vi "Event Receive.vi"(11 "jettl Event Actor in":refnum<class "jettl Event Actor.lvclass">) -> (2 "Event Msg":refnum<user-event>, 3 "jettl Event Actor out":refnum<class "jettl Event Actor.lvclass">)   [LabVIEW 2021, in "jettl.lvlib" / "jettl Event Actor.lvclass"]
uses:
  jettl Event Actor.lvclass
  Actor/Msg/Msg.lvclass
  jettl Event Actor.lvclass/jettl Event Actor.ctl
  jettl.lvlib
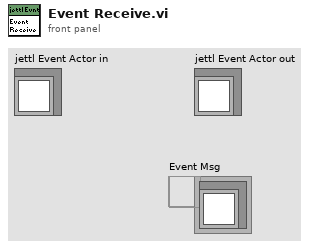
[diagram p1: front panel]
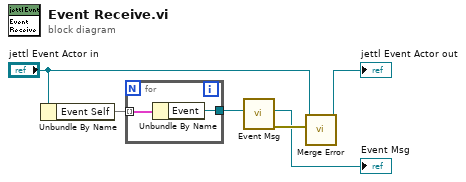
[diagram p0: block diagram]
diagram:
  n1 = Unbundle By Name("jettl Event Actor in") -> ("Event Self"=w4:map{string, refnum<data-value>})
  n2 = for {
    tunnel: w4 -> [w8] mode=indexing
    tunnel: [w7] -> w3
    n3 = Unbundle By Name(w8) -> ("Event"=w7:refnum<data-value>)
  }
  n4 = call "Event Msg.vi"("Event"=w3) -> ("error out"=w2:errorcluster, "Event Msg"=→"Event Msg":refnum<user-event>)  [unwired: 9 in]
  n5 = call-dynamic "Merge Error.vi"("Error"=w2, "Set Error in"="jettl Event Actor in") -> ("Set Error out"=→"jettl Event Actor out":refnum<class "jettl Event Actor.lvclass">)  [unwired: 9 in]
